vi "SV Set Parent Values.vi"(0 "child class in":refnum<class "SV Signal.lvclass">, 5 "parent class":refnum<class "SV Signal.lvclass">, 11 "error in (no error)":errorcluster) -> (4 "child class out":refnum<class "SV Signal.lvclass">, 15 "error out":errorcluster)   [LabVIEW 2017, in "SV Signal.lvclass"]
uses:
  <vilib>/addons/_NISVFA/_Generation/Signal Generation/SV Signal/SV Signal.lvclass
  <vilib>/addons/_NISVFA/_Generation/Signal Generation/SV Signal/SV Signal.lvclass/SV Signal.ctl
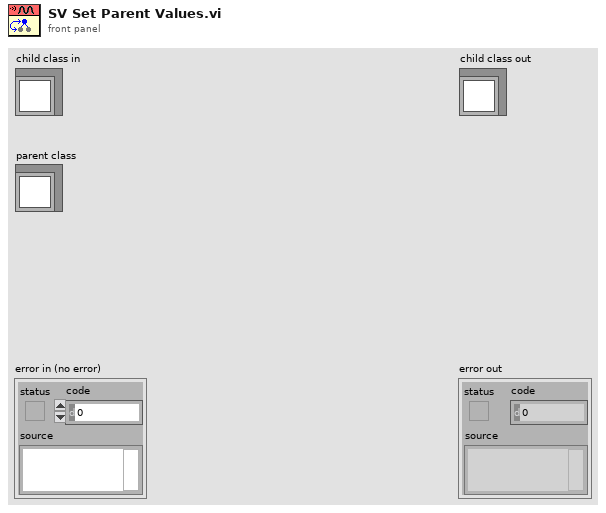
[diagram p1: front panel]
types:
  T1 = typedef "SV Signal.lvclass/sv_System Timing Model.ctl" = i64
  T2 = cluster{"profile":enum16{"Linear", "Half cosine"}, "durations [s]":cluster{"ramp-up":dbl, "transition":dbl, "ramp-down":dbl}}
  T3 = typedef "SV Signal.lvclass/sv_Generation State.ctl" = enum16{"Idle", "Ramp Up", "Pre-Measurement Settling", "Measurement", "Post-Measurement Settling", "Discrete Sweep Transition", "Ramp Down", "Update"}
  T4 = cluster{"RESET":bool, "generator timestamp":timestamp, "elapsed seconds":dbl, "elapsed samples":u64, "generation state":T3, "time offset at state":dbl, "samples generated at state":u64, "signal state":variant}
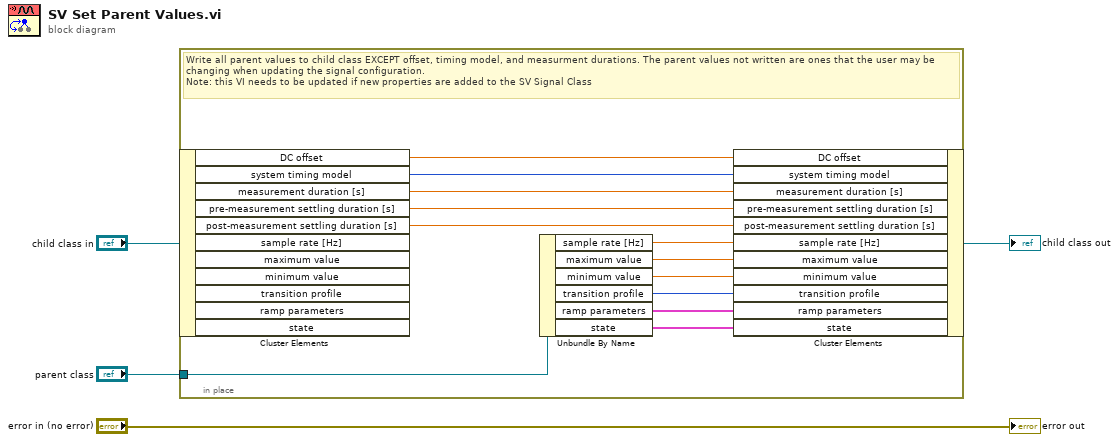
[diagram p0: block diagram]
diagram:
  n1 = in-place {
    in-place-border: "parent class" -> [w16]
    # "Write all parent values to child class EXCEPT offset, timing model, and measurment durations. The parent values not written are ones that the user may be changing when updating the signal configuration. \nNote: this VI needs to be updated if new properties are added to the SV Signal Class"
    n2 = in-place-cluster #1("child class in") -> ("DC offset"=w9:dbl, "system timing model"=w8:T1, "measurement duration [s]"=w7:dbl, "pre-measurement settling duration [s]"=w6:dbl, "post-measurement settling duration [s]"=w5:dbl)  [unwired: 6 out]
    n3 = Unbundle By Name(w16) -> ("sample rate [Hz]"=w15:dbl, "maximum value"=w14:dbl, "minimum value"=w13:dbl, "transition profile"=w12:enum16{"Immediate", "Next optimum", "Ramp"}, "ramp parameters"=w11:T2, "state"=w10:T4)
    n4 = in-place-cluster #1("DC offset"=w9, "system timing model"=w8, "measurement duration [s]"=w7, "pre-measurement settling duration [s]"=w6, "post-measurement settling duration [s]"=w5, "sample rate [Hz]"=w15, "maximum value"=w14, "minimum value"=w13, "transition profile"=w12, "ramp parameters"=w11, "state"=w10) -> (→"child class out":refnum<class "SV Signal.lvclass">)
  }
  "error out" <- "error in (no error)"
